vi "XML_Get Child Nodes[].vi"(8 "错误输入（无错误）":errorcluster, 11 "ref in":refnum<k20>) -> (0 "错误输出":errorcluster, 1 "NodeNames[]":string[](array[string]), 2 "ElementChildNod[]":refnum<k20>[](array[refnum]), 3 "ref out":refnum<k20>)   [LabVIEW 2016]
uses:
  <resource>/objmgr/DOMUserDefRef.rc
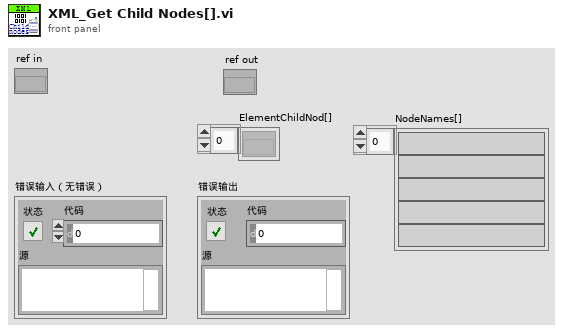
[diagram p1: front panel]
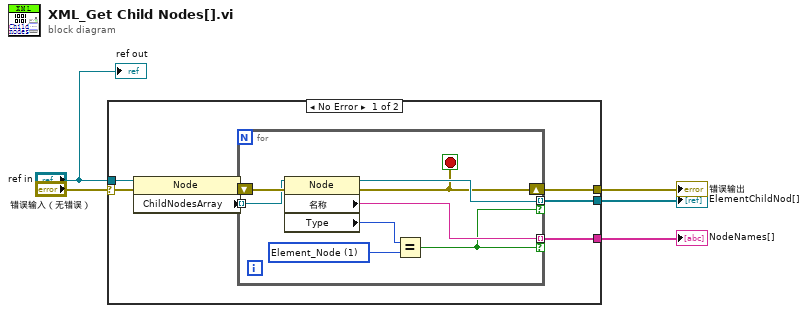
[diagram p0: block diagram]
diagram:
  n1 = case shown="No Error" "错误输入（无错误）" {
    selector: "错误输入（无错误）" -> [w11 w21]
    tunnel: "ref in" -> [w12 _]
    tunnel: [w8 _] -> w4
    tunnel: [w7 w21] -> w3
    tunnel: [w6 _] -> w2
    frame No Error {
      n2 = property on="属性节点" class="Node"(reference=w12, error in=w11) -> (error out=w9:errorcluster, "ChildNodesArray"=w10:refnum<k20>[])  [unwired: 1 out]
      n3 = for {
        tunnel: w10 -> [w19] mode=indexing
        shift-right: [w16] -> w7
        shift-left: w9 -> [w20]
        tunnel: [w17] -> w8 mode=indexing if=w13
        tunnel: [w14] -> w6 mode=indexing if=w13
        stop <- w16 stop-if-true
        w18 = 1 items=["Element_Node"=1, "Attribute_Node"=2, "Text_Node"=3, "CDATASection_Node"=4, "EntityReference_Node"=5, "Entity_Node"=6, "ProcessingInstruction_Node"=7, "Comment_Node"=8, "Document_Node"=9, "DocumentType_Node"=10, "DocumentFragment_Node"=11, "Notation_Node"=12] ("节点类型")
        n4 = property on="属性节点" class="Node"(reference=w19, error in=w20) -> (reference out=w17:refnum<k20>, error out=w16:errorcluster, "名称"=w14:string, "Type"=w15:i32)
        n5 = Equal?(x=w15, y=w18) -> (x = y?=w13:bool)
      }
    }
    frame Error {
    }
  }
  "错误输出" <- w3
  "ElementChildNod[]" <- w4
  "NodeNames[]" <- w2
  "ref out" <- "ref in"
